vi "Absolute Move.vi"(7 "Target position":dbl, 9 "Connection Cluster in":T1) -> (3 "Connection Cluster out":T1)   [LabVIEW 2020]
doc: "Set Absolute Position Move to start."
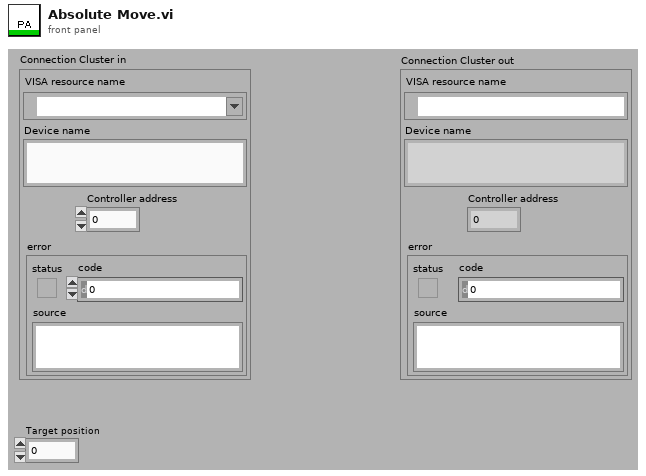
[diagram p1: front panel]
types:
  T1 = cluster{"VISA resource name":refnum<visa-resource-name>, "Device name":string, "Controller address":i32, "error":errorcluster}
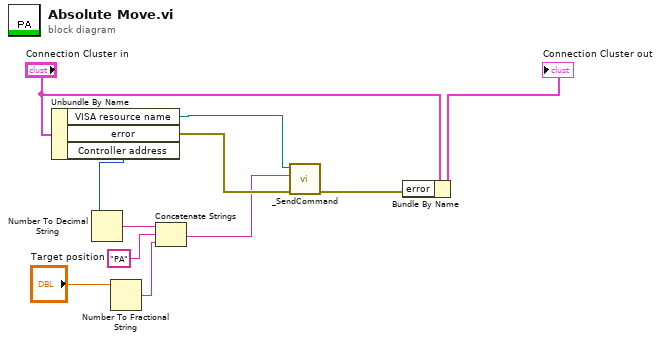
[diagram p0: block diagram]
diagram:
  n1 = Unbundle By Name("Connection Cluster in") -> ("VISA resource name"=w3:refnum<visa-resource-name>, "error"=w4:errorcluster, "Controller address"=w2:i32)
  n2 = Number To Decimal String(number=w2) -> (decimal integer string=w11:string)  [unwired: 1 out]
  n3 = Number To Fractional String(number="Target position") -> (F-format string=w8:string)  [unwired: 3 out]
  n4 = Concatenate Strings(w11, "PA" ("strCommand"), w8) -> (w1:string)
  n5 = call "_SendCommand.vi"("error in"=w4, "Command"=w1, "Instrument Channel"=w3) -> ("error out"=w7:errorcluster)  [unwired: 7 in, 1 out]
  n6 = Bundle By Name(cluster="Connection Cluster in", "error"=w7) -> (→"Connection Cluster out":T1)
